vi "Transducer Calibration Global.vi"(8 "Action":T2, 9 "Vref In":dbl, 10 "Sensor":T3, 11 "Data In":T1[](array[typedef])) -> (1 "Vref (5V Nominal)":dbl, 2 "Calibration Data":T1={"Scale"=1.0, "Offset"=0.0})   [LabVIEW 2015]
uses:
  Sensor Enum.ctl
  Transducer Calibration Global Action.ctl
  Transducer Calibration Control.ctl
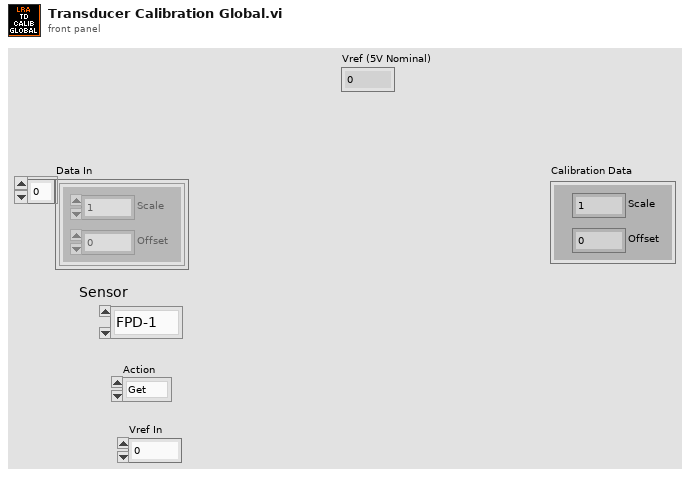
[diagram p1: front panel]
types:
  T1 = typedef "Transducer Calibration Control.ctl" = cluster{"Scale":dbl, "Offset":dbl}
  T2 = typedef "Transducer Calibration Global Action.ctl" = enum16{"Get", "Set"}
  T3 = typedef "Sensor Enum.ctl" = enum16{"FPD-1", "FPD-2", "FPD-3", "OPD-1", "OPD-2", "OPD-3", "AP-1", "PC-1", "PC-2", "VBAT", "VCOMP", "ICOMP", "TC-1", "TC-COMP"}
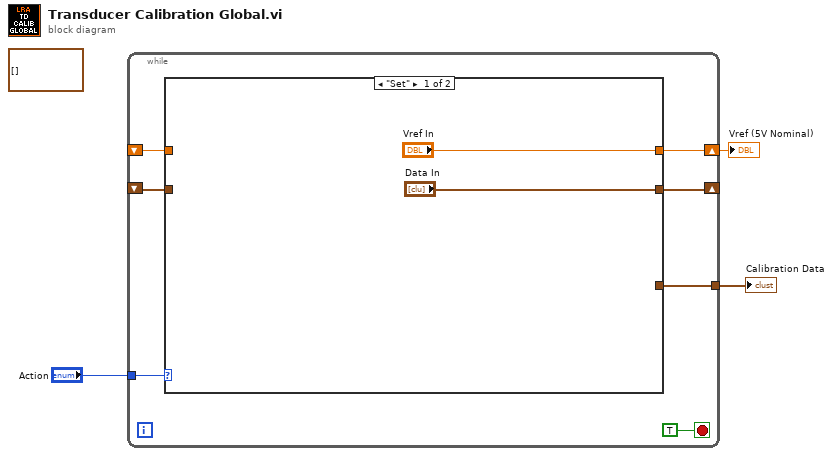
[diagram p0: block diagram]
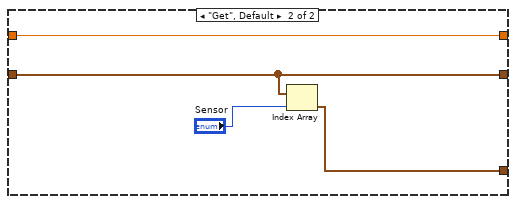
[diagram p2: hidden frame]
diagram:
  (unwired) T1[] []
  n1 = while {
    tunnel: "Action" -> [w9]
    shift-right: [w8] -> _
    shift-left: _ -> [w6]
    tunnel: [w7] -> w2
    shift-right: [w5] -> w1
    shift-left: _ -> [w4]
    stop <- TRUE stop-if-true
    n2 = case shown="\"Set\"" w9 {
      tunnel: ["Data In" w14] -> w8
      tunnel: [_ w15] -> w7
      tunnel: w6 -> [_ w14]
      tunnel: ["Vref In" w13] -> w5
      tunnel: w4 -> [_ w13]
      frame "Set" {
      }
      frame "Get", Default {
        n3 = Index Array(array=w14, index="Sensor") -> (element=w15:T1)
      }
    }
  }
  "Calibration Data" <- w2
  "Vref (5V Nominal)" <- w1
